vi "Point in Polygon.vi"(8 "polyY":dbl[](array[numeric]), 9 "polyX":dbl[](array[numeric]), 10 "y":dbl, 11 "x":dbl) -> (3 "Inside?":bool)   [LabVIEW 2021]
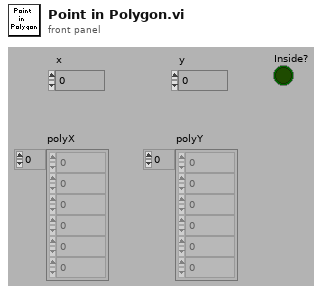
[diagram p1: front panel]
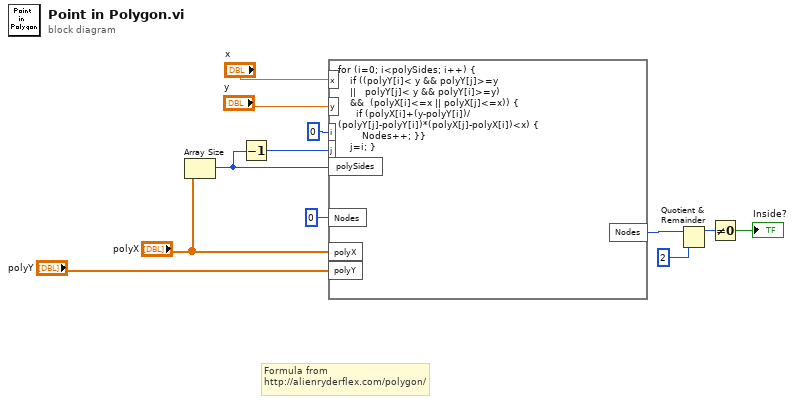
[diagram p0: block diagram]
diagram:
  # "Formula from\nhttp://alienryderflex.com/polygon/"
  n1 = Array Size(array="polyX") -> (size(s)=w7:i32)
  n2 = Decrement(x=w7) -> (x-1=w6:i32)
  n3 = formula code="for (i=0; i<polySides; i++) {\n    if ((polyY[i]< y && polyY[j]>=y\n    ||   polyY[j]< y && polyY[i]>=y)\n    &&  (polyX[i]<=x || polyX[j]<=x)) {\n      if (polyX[i]+(y-polyY[i])/(polyY[j]-polyY[i])*(polyX[j]-polyX[i])<x) {\n        Nodes++; }}\n    j=i; }"("i"=i16 0 ("input variable"), "j"=w6, "polySides"=w7, "Nodes"=i16 0 ("input variable"), "polyX"="polyX", "polyY"="polyY", "x"="x", "y"="y") -> ("Nodes"=w10:i16)
  n4 = Quotient & Remainder(x=w10, y=i16 2) -> (x-y*floor(x/y)=w9:i16)  [unwired: 1 out]
  n5 = Not Equal To 0?(x=w9) -> (x != 0?=→"Inside?":bool)
